vi "StartICL.vi"(8 "error in (no error)":errorcluster, 11 "DeviceManager in":refnum<class "DeviceManager.lvclass">) -> (0 "error out":errorcluster, 3 "DeviceManager out":refnum<class "DeviceManager.lvclass">)   [LabVIEW 2023, in "DeviceManager.lvclass"]
uses:
  DeviceManager.lvclass
  DeviceManager.lvclass/DeviceManager.ctl
  <vilib>/JKI/JKI DotNet System Exec/dotnet_system_exec/dotnet_system_exec.lvclass
panel:
  out "StdErr":string
  out "StdOut":string
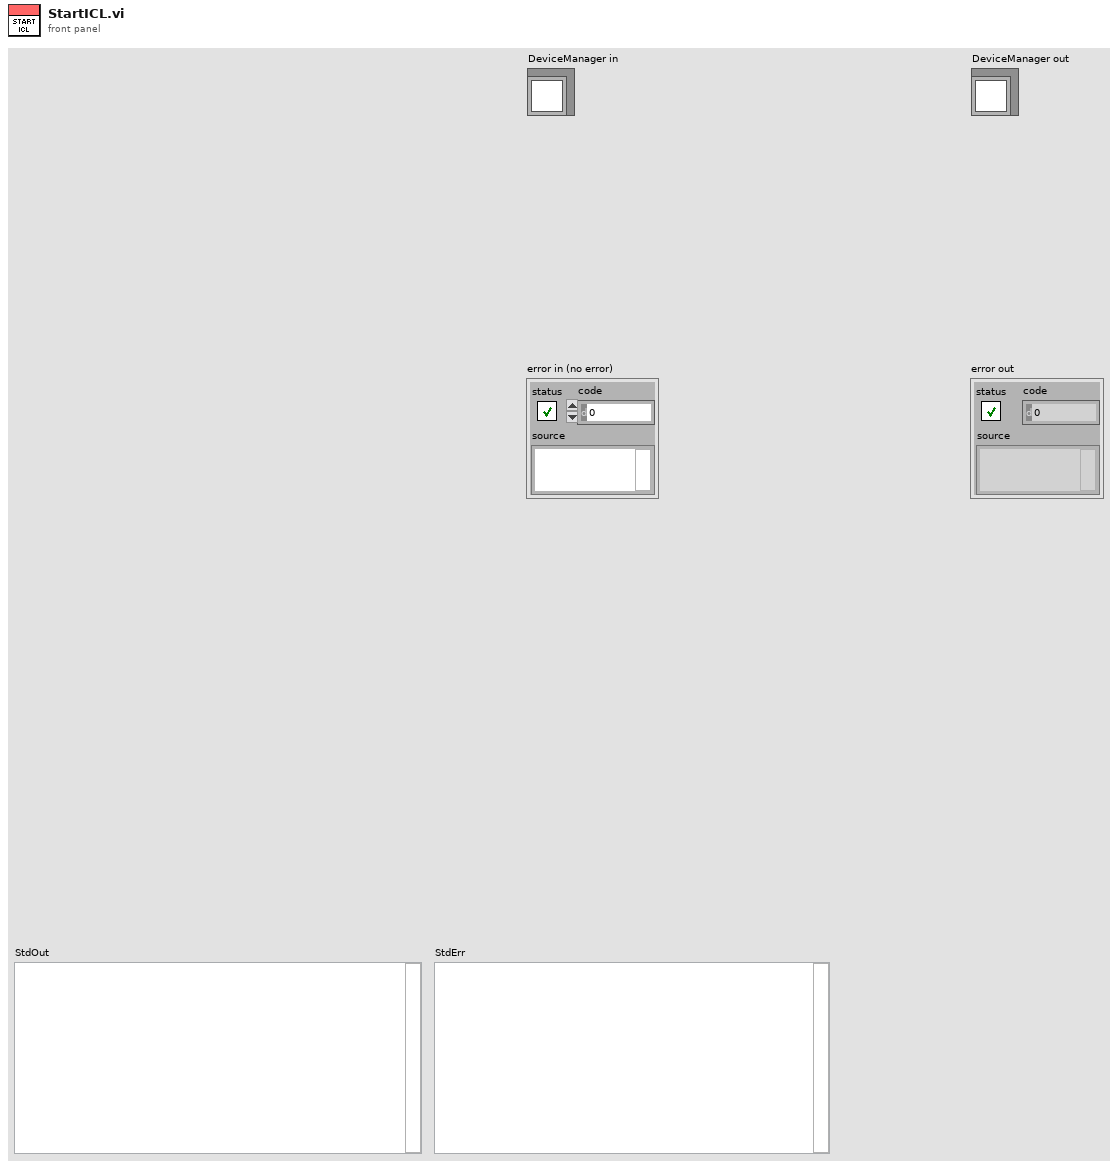
[diagram p1: front panel]
types:
  T1 = cluster{"stdout event":refnum<user-event>, "stderr event":refnum<user-event>, "process_exit event":refnum<user-event>}
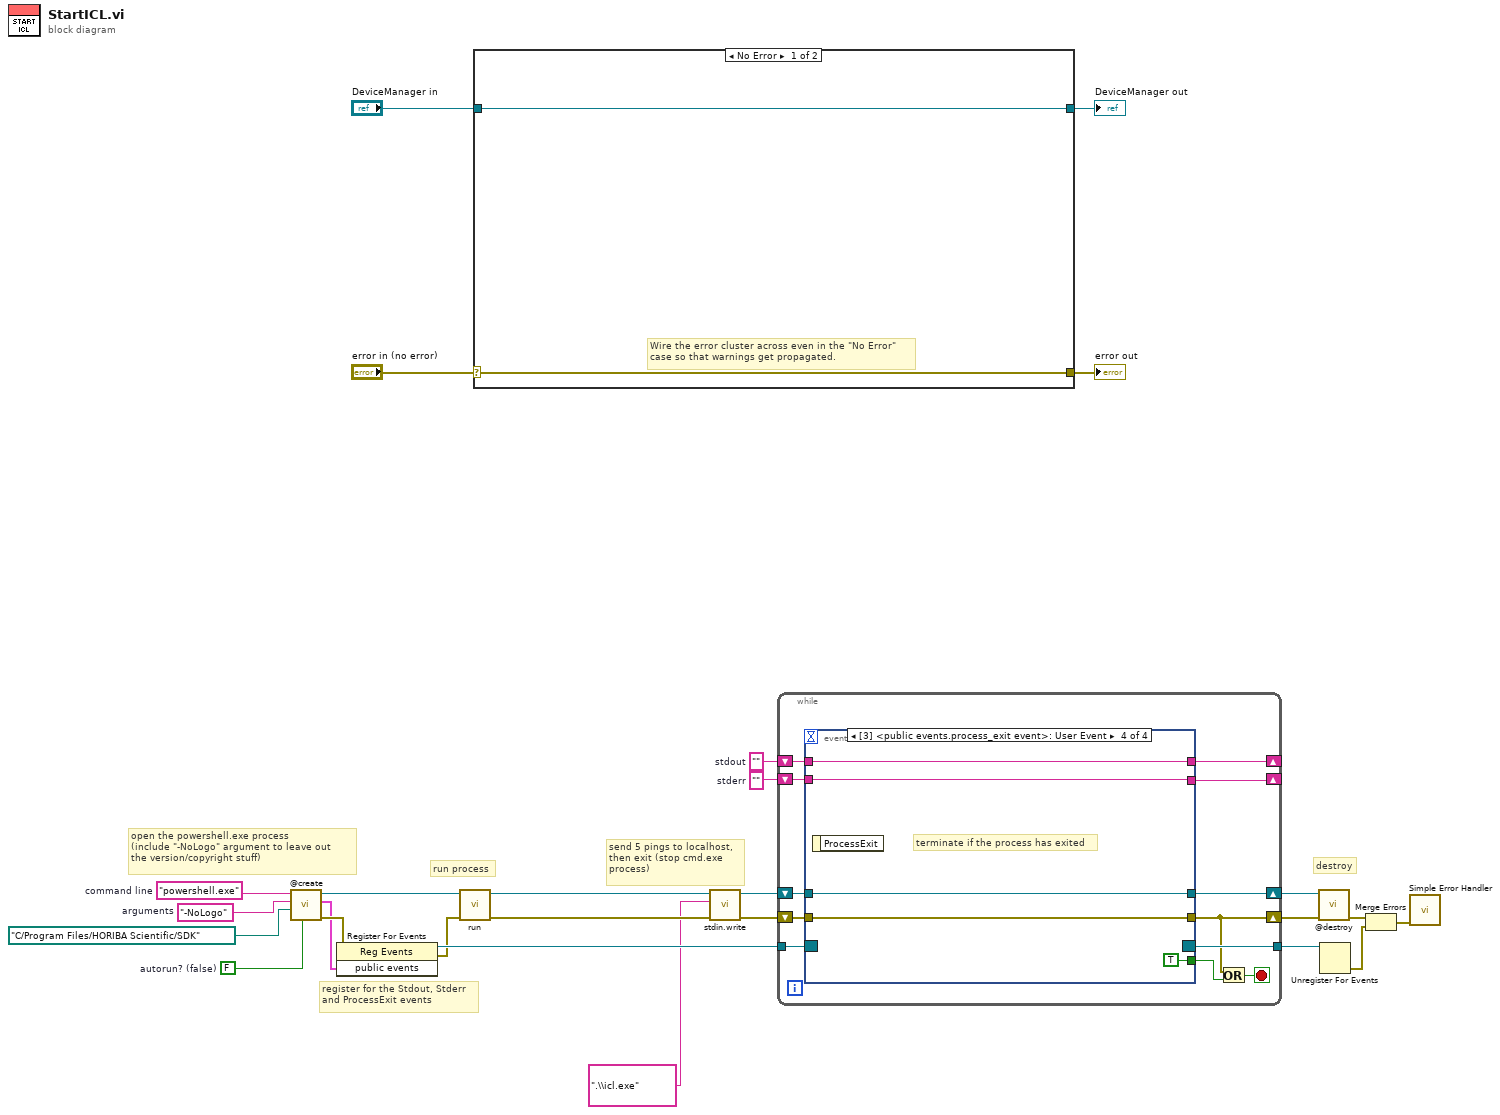
[diagram p0: block diagram]
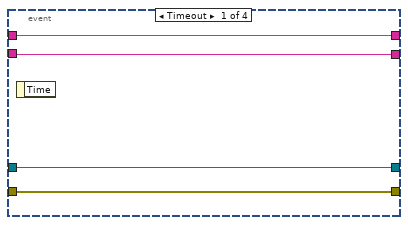
[diagram p2: hidden frame]
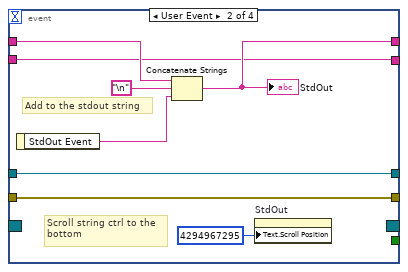
[diagram p3: hidden frame]
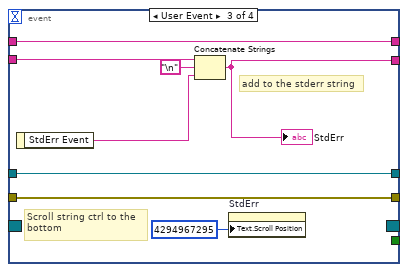
[diagram p4: hidden frame]
diagram:
  w1 = FALSE  # autorun? (false)
  w3 = "-NoLogo"  # arguments
  w4 = "powershell.exe"  # command line
  w10 = ""  # stderr
  w14 = ""  # stdout
  # "send 5 pings to localhost,\nthen exit (stop cmd.exe \nprocess)"
  # "destroy"
  # "register for the Stdout, Stderr \nand ProcessExit events"
  # "run process"
  # "open the powershell.exe process\n(include \"-NoLogo\" argument to leave out\nthe version/copyright stuff)"
  n1 = call <vilib>:"@create.vi"("autorun? (false)"=w1, "working directory (c:\\)"=path "C:/Program Files/HORIBA Scientific/SDK" ("working directory"), "arguments (\"\")"=w3, "command line (cmd.exe)"=w4) -> ("error out"=w13:errorcluster, "public events"=w11:T1, "dotnet_system_exec out"=w21:refnum<class "dotnet_system_exec.lvclass">)  [unwired: 5 in]
  n2 = register-events(error in=w13, w11) -> (reference out=w20:refnum<event-registration>, error out=w12:errorcluster)  [unwired: 1 in]
  n3 = call <vilib>:"run.vi"("error in (no error)"=w12, "dotnet_system_exec in"=w21) -> ("error out"=w8:errorcluster, "dotnet_system_exec out"=w9:refnum<class "dotnet_system_exec.lvclass">)  [unwired: 8 in]
  n4 = case shown="No Error" "error in (no error)" {
    selector: "error in (no error)" -> [w27 w30]
    tunnel: [w27 w30] -> w25
    tunnel: [w28 w29] -> w23
    tunnel: "DeviceManager in" -> [w28 w29]
    frame No Error {
      # "Wire the error cluster across even in the \"No Error\"\ncase so that warnings get propagated."
    }
    frame Error {
    }
  }
  "error out" <- w25
  "DeviceManager out" <- w23
  n5 = call-dynamic "stdin.write.vi"("error in (no error)"=w8, "stdin"=".\\icl.exe", "dotnet_system_exec in"=w9) -> ("error out"=w6:errorcluster, "dotnet_system_exec out"=w7:refnum<class "dotnet_system_exec.lvclass">)  [unwired: 7 in]
  n6 = while {
    shift-right: [w42] -> w22
    shift-left: w7 -> [w41]
    shift-right: [w33] -> w18
    shift-left: w6 -> [w40]
    tunnel: w20 -> [w39]
    tunnel: [w38] -> w19
    shift-right: [w36] -> _
    shift-left: w14 -> [w37]
    shift-right: [w34] -> _
    shift-left: w10 -> [w35]
    stop <- w32 stop-if-true
    n7 = event shown="[3] <public events.process_exit event>: User Event" {
      selector: w39 -> [_ _ _ _]
      dyn-events: [_ _ _ _] -> w38
      timeout: _ -> [_ _ _ _]
      tunnel: [w46 w54 w62 w65] -> w42
      tunnel: w41 -> [w46 w54 w62 w65]
      tunnel: w40 -> [w45 w53 w61 w64]
      tunnel: [w45 w53 w61 w64] -> w33
      tunnel: w37 -> [w44 w50 w57 w66]
      tunnel: [w44 w51 w57 w66] -> w36
      tunnel: [_ _ _ TRUE ("ProcessExit")] -> w31
      tunnel: w35 -> [w43 w48 w58 w67]
      tunnel: [w43 w48 w56 w67] -> w34
      event Timeout {
        n8 = event-data() -> ()  [unwired: 1 in, 1 out]
      }
      event User Event {
        # "Scroll string ctrl to the \nbottom"
        # "Add to the stdout string"
        n9 = event-data() -> ("StdOut Event"=w49:string)  [unwired: 1 in]
        n10 = Concatenate Strings(w50, "\n", w49) -> (w51:string)
        "StdOut" <- w51
        n11 = property on="StdOut" class="Str"("Text.Scroll Position"=u32 4294967295) -> ()  [unwired: 2 in, 2 out]
      }
      event User Event {
        # "Scroll string ctrl to the \nbottom"
        # "add to the stderr string"
        n12 = event-data() -> ("StdErr Event"=w59:string)  [unwired: 1 in]
        n13 = Concatenate Strings(w58, "\n", w59) -> (w56:string)
        "StdErr" <- w56
        n14 = property on="StdErr" class="Str"("Text.Scroll Position"=u32 4294967295) -> ()  [unwired: 2 in, 2 out]
      }
      event User Event {
        # "terminate if the process has exited"
        n15 = event-data() -> ()  [unwired: 1 in, 1 out]
      }
    }
    n16 = Or(x=w33, y=w31) -> (x .or. y?=w32:bool)
  }
  n17 = call-dynamic "@destroy.vi"("error in (no error)"=w18, "dotnet_system_exec in"=w22) -> ("error out"=w17:errorcluster)  [unwired: 8 in, 1 out]
  n18 = Unregister For Events(event registration refnum=w19) -> (error out=w16:errorcluster)  [unwired: 1 in]
  n19 = Merge Errors(w17, w16) -> (w15:errorcluster)
  n20 = call <vilib>:"Simple Error Handler.vi"("error in (no error)"=w15) -> ()  [unwired: 4 in, 5 out]
